vi "rs3_RGB_to_Picture7.vi"(0 "RGB array":u8[](array[numeric])=array[921600 elements], 1 "Color format":enum16{"Monochrome", "RGB internal (RGB)"}(ring), 2 "ROI on":bool, 3 "ROI reduction 1/x":i32=10, 5 "RGB  X, width":i32=1280, 7 "RGB Y, height":i32=720, 9 "AWB":bool, 11 "error in (no error)":errorcluster, 12 "White Balance":T1={"Red"=1.0, "Green"=1.0, "Blue"=1.0, "Gain"=2.0} {"Gain" format="%_3g"; "Blue" format="%_3g"; "Green" format="%_3g"; "Red" format="%_3g"}, 14 "White Balance":bool) -> (6 "new picture":picture, 15 "error out":errorcluster)   [LabVIEW 2017, in "libRealSense3.lvlib"]
doc: "This converts an 1D input array into a 2D picture, and applies some white balance correction if requested."
uses:
  libRealSense3.lvlib
  <vilib>/Analysis/baseanly.llb/Mean (DBL).vi
  <vilib>/Analysis/NI_AALBase.lvlib
panel:
  # "RS3 RGB to Picture 5"
  # "(C) Intel Corp. 2017,  AGJ"
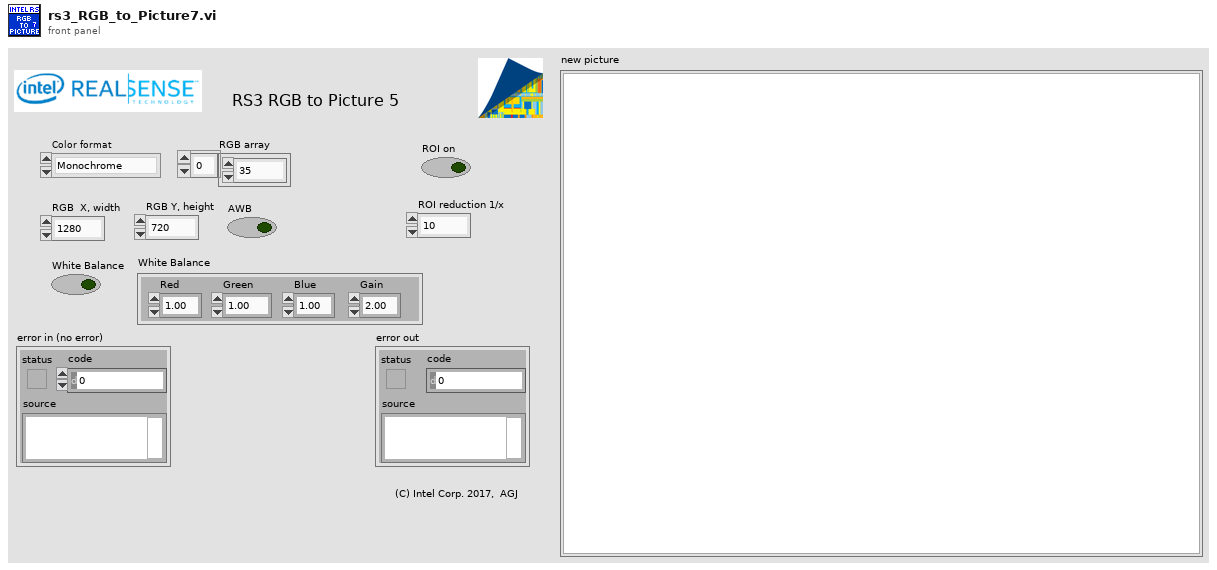
[diagram p1: front panel]
types:
  T1 = cluster{"Red":dbl, "Green":dbl, "Blue":dbl, "Gain":dbl}
  T2 = typedef "imagedata.ctl" = cluster{"image type":i32, "image depth":i32, "image":u8[], "mask":u8[], "colors":u32[], "Rectangle":cluster{"left":i16, "top":i16, "right":i16, "bottom":i16}}
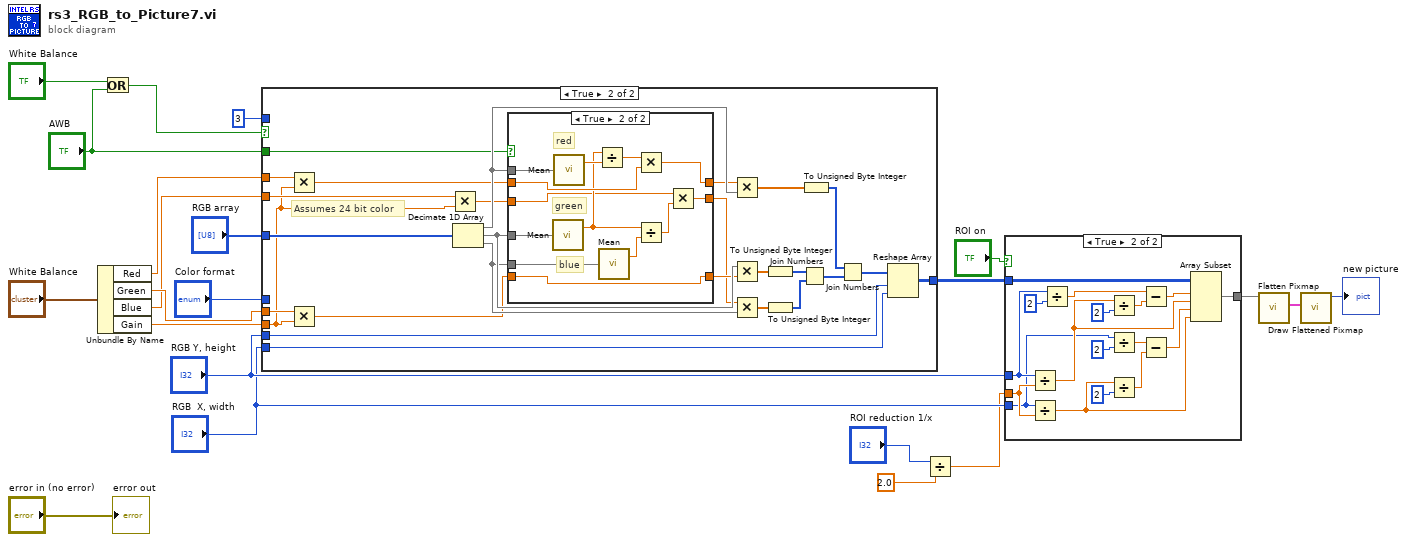
[diagram p0: block diagram]
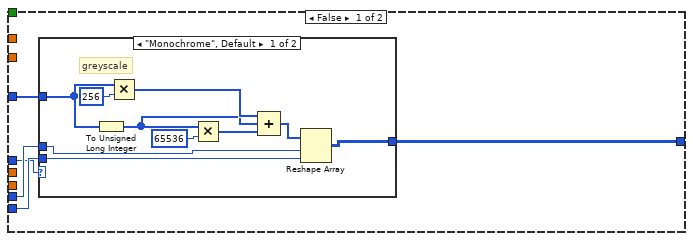
[diagram p3: hidden frame]
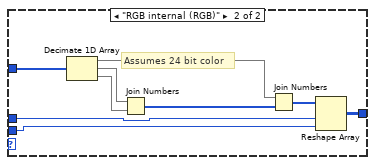
[diagram p4: hidden frame]
diagram:
  n1 = Unbundle By Name("White Balance") -> ("Red"=w20:dbl, "Green"=w19:dbl, "Blue"=w18:dbl, "Gain"=w11:dbl)
  n2 = Or(x="White Balance", y="AWB") -> (x .or. y?=w13:bool)
  n3 = case shown="True" w13 {
    tunnel: "RGB array" -> [w27 w70]
    tunnel: "RGB Y, height" -> [w26 w49]
    tunnel: "RGB  X, width" -> [w25 w48]
    tunnel: 3 ("# of bytes/number") -> [_ _]
    tunnel: w20 -> [_ w56]
    tunnel: w19 -> [_ w54]
    tunnel: w18 -> [_ w52]
    tunnel: "AWB" -> [_ w57]
    tunnel: "Color format" -> [w24 _]
    tunnel: w11 -> [_ w50]
    tunnel: [w23 w47] -> w7
    frame False {
      n4 = case shown="\"Monochrome\", Default" w24 {
        tunnel: [w35 w45] -> w23
        tunnel: w27 -> [w31 w43]
        tunnel: w26 -> [w37 w42]
        tunnel: w25 -> [w36 w41]
        frame "Monochrome", Default {
          # "greyscale"
          n5 = To Unsigned Long Integer(number=w31) -> (unsigned 32bit integer=w28:u32[])
          n6 = Multiply(x=w31, y=u32 256) -> (x*y=w32:u32[])
          n7 = Multiply(x=w28, y=u32 65536) -> (x*y=w30:u32[])
          n8 = Compound Arithmetic op=ADD(w32, w28, w30) -> (w29:u32[])
          n9 = Reshape Array(w29, w37, w36) -> (w35:u32[][])
        }
        frame "RGB internal (RGB)" {
          # "Assumes 24 bit color"
          n10 = Decimate 1D Array(w43) -> (w40:u8[], w39:u8[], w38:u8[])
          n11 = Join Numbers(hi=w39, lo=w38) -> ((hi.lo)=w46:u16[])
          n12 = Join Numbers(hi=w40, lo=w46) -> ((hi.lo)=w44:u32[])
          n13 = Reshape Array(w44, w42, w41) -> (w45:u32[][])
        }
      }
    }
    frame True {
      # "Assumes 24 bit color"
      n14 = Multiply(x=w56, y=w50) -> (x*y=w55:dbl)
      n15 = Multiply(x=w54, y=w50) -> (x*y=w53:dbl)
      n16 = Multiply(x=w52, y=w50) -> (x*y=w51:dbl)
      n17 = Decimate 1D Array(w70) -> (w63:u8[], w62:u8[], w61:u8[])
      n18 = case shown="True" w57 {
        tunnel: w63 -> [_ w88]
        tunnel: w62 -> [_ w87]
        tunnel: w61 -> [_ w86]
        tunnel: [w75 w81] -> w60
        tunnel: w55 -> [w75 w82]
        tunnel: [w74 w76] -> w59
        tunnel: w53 -> [w74 w76]
        tunnel: w51 -> [w73 w78]
        tunnel: [w73 w77] -> w58
        frame False {
        }
        frame True {
          # "blue"
          # "green"
          # "red"
          n19 = call-poly <vilib>:"Mean.vi"("X"=w87) -> ("mean"=w80:dbl)  [unwired: 1 out]
          n20 = call-poly <vilib>:"Mean.vi"("X"=w88) -> ("mean"=w85:dbl)  [unwired: 1 out]
          n21 = Divide(x=w80, y=w85) -> (x/y=w83:dbl)
          n22 = call-poly <vilib>:"Mean.vi"("X"=w86) -> ("mean"=w84:dbl)  [unwired: 1 out]
          n23 = Multiply(x=w83, y=w82) -> (x*y=w81:dbl)
          n24 = Divide(x=w80, y=w84) -> (x/y=w79:dbl)
          n25 = Multiply(x=w78, y=w79) -> (x*y=w77:dbl)
        }
      }
      n26 = Multiply(x=w60, y=w63) -> (x*y=w69:dbl[])
      n27 = Multiply(x=w62, y=w59) -> (x*y=w65:dbl[])
      n28 = Multiply(x=w58, y=w61) -> (x*y=w66:dbl[])
      n29 = To Unsigned Byte Integer(number=w65) -> (unsigned 8bit integer=w67:u8[])
      n30 = To Unsigned Byte Integer(number=w66) -> (unsigned 8bit integer=w64:u8[])
      n31 = Join Numbers(hi=w67, lo=w64) -> ((hi.lo)=w72:u16[])
      n32 = To Unsigned Byte Integer(number=w69) -> (unsigned 8bit integer=w68:u8[])
      n33 = Join Numbers(hi=w68, lo=w72) -> ((hi.lo)=w71:u32[])
      n34 = Reshape Array(w71, w49, w48) -> (w47:u32[][])
    }
  }
  n35 = Divide(x="ROI reduction 1/x", y=2.0) -> (x/y=w1:dbl)
  n36 = case shown="True" "ROI on" {
    tunnel: w1 -> [_ w91]
    tunnel: w7 -> [w89 w94]
    tunnel: [w89 w93] -> w6
    tunnel: "RGB Y, height" -> [_ w92]
    tunnel: "RGB  X, width" -> [_ w90]
    frame False {
    }
    frame True {
      n37 = Divide(x=w92, y=w91) -> (x/y=w100:dbl)
      n38 = Divide(x=w90, y=w91) -> (x/y=w98:dbl)
      n39 = Divide(x=w92, y=2) -> (x/y=w102:dbl)
      n40 = Divide(x=w100, y=2) -> (x/y=w103:dbl)
      n41 = Divide(x=w90, y=2) -> (x/y=w97:dbl)
      n42 = Divide(x=w98, y=2) -> (x/y=w96:dbl)
      n43 = Subtract(x=w102, y=w103) -> (x-y=w101:dbl)
      n44 = Subtract(x=w97, y=w96) -> (x-y=w95:dbl)
      n45 = Array Subset(array=w94, index (row)=w101, length (row)=w100, index (col)=w95, length (col)=w98) -> (w93:u32[][])
    }
  }
  n46 = call <vilib>:"Flatten Pixmap.vi"("24-bit pixmap"=w6) -> ("image data"=w10:T2)  [unwired: 10 in]
  n47 = call <vilib>:"Draw Flattened Pixmap.vi"("image data"=w10) -> ("new picture"=→"new picture":picture)  [unwired: 8 in]
  "error out" <- "error in (no error)"
